vi "main_receiver_MIMO_OFDM.vi"() -> ()   [LabVIEW 2020] (continued)
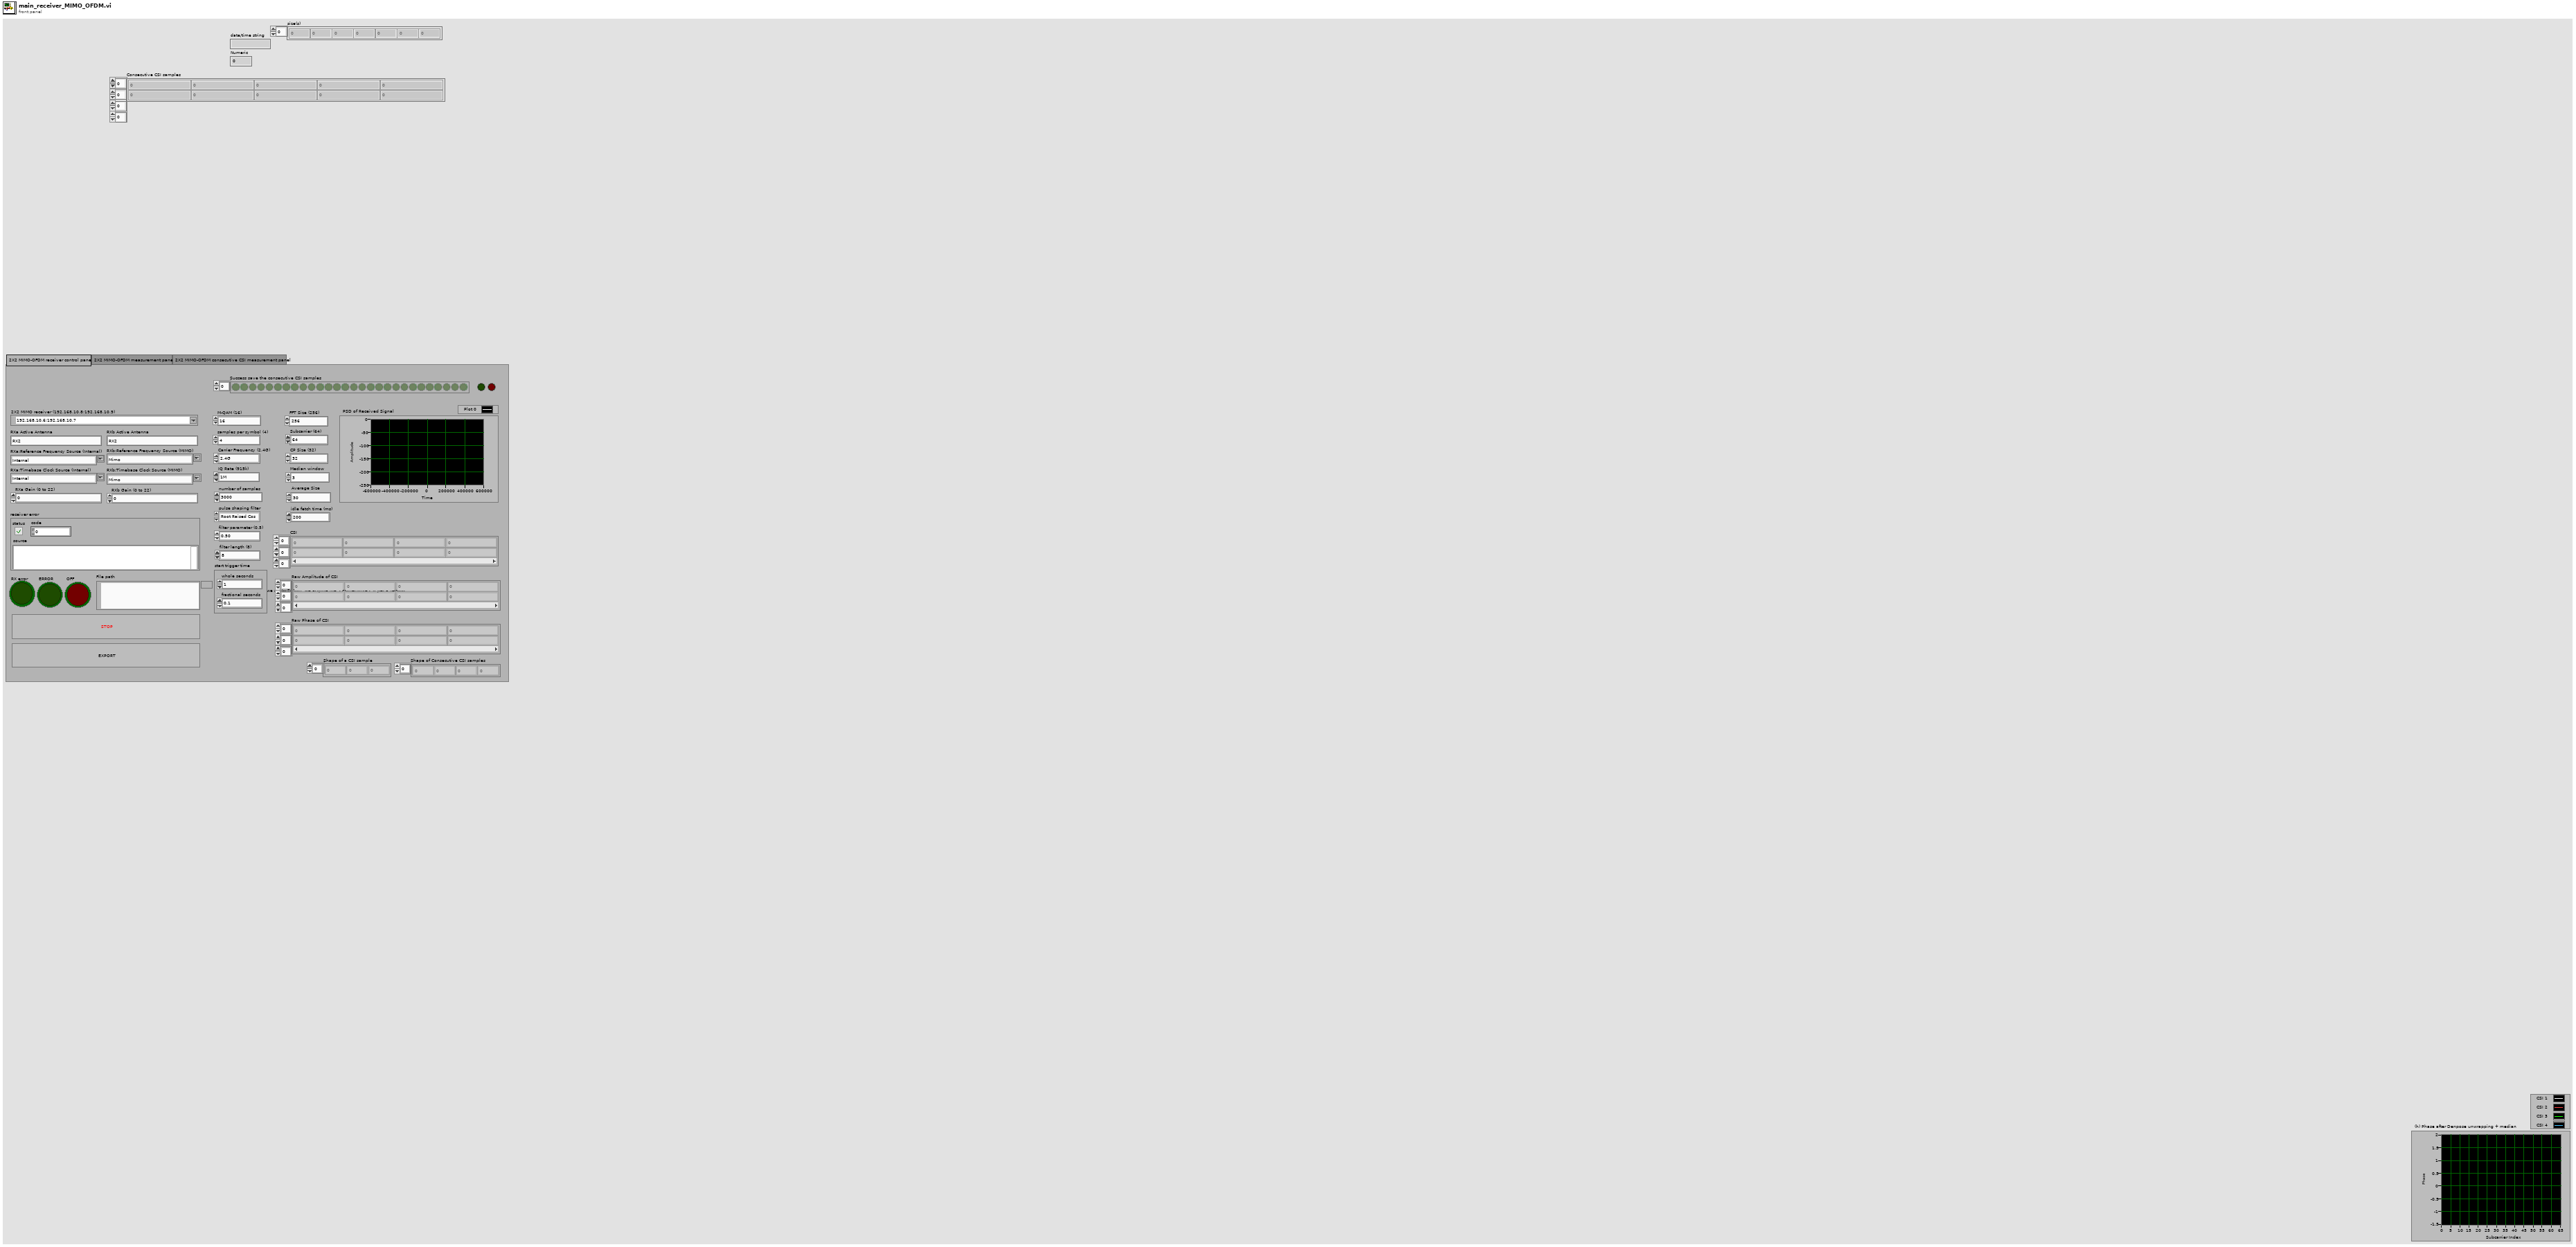
[diagram p1: front panel]
types:
  T1 = enum32{"2X2 MIMO-OFDM receiver control panel", "2X2 MIMO-OFDM measurement panel", "2X2 MIMO-OFDM consecutive CSI measurement panel"}
  T2 = typedef "niUSRP Timestamp.ctl" = cluster{"whole seconds":u64, "fractional seconds":dbl}
  T3 = enum16{"none", "Raised Cosine", "Root Raised Cos", "Gaussian"}
  T4 = enum16{"FSK", "PSK", "QAM", "MSK", "PAM", "ASK", "CPM"}
  T5 = cluster{"samples per symbol (16)":i32, "symbol map":cdb[]}
  T6 = typedef "niAMT.lvlib/Complex Data Waveform.ctl" = cluster{"t0":dbl, "dt":dbl, "Y":cdb[]}
  T7 = cluster{"f0":dbl, "df":dbl, "imaginary part":dbl[]}
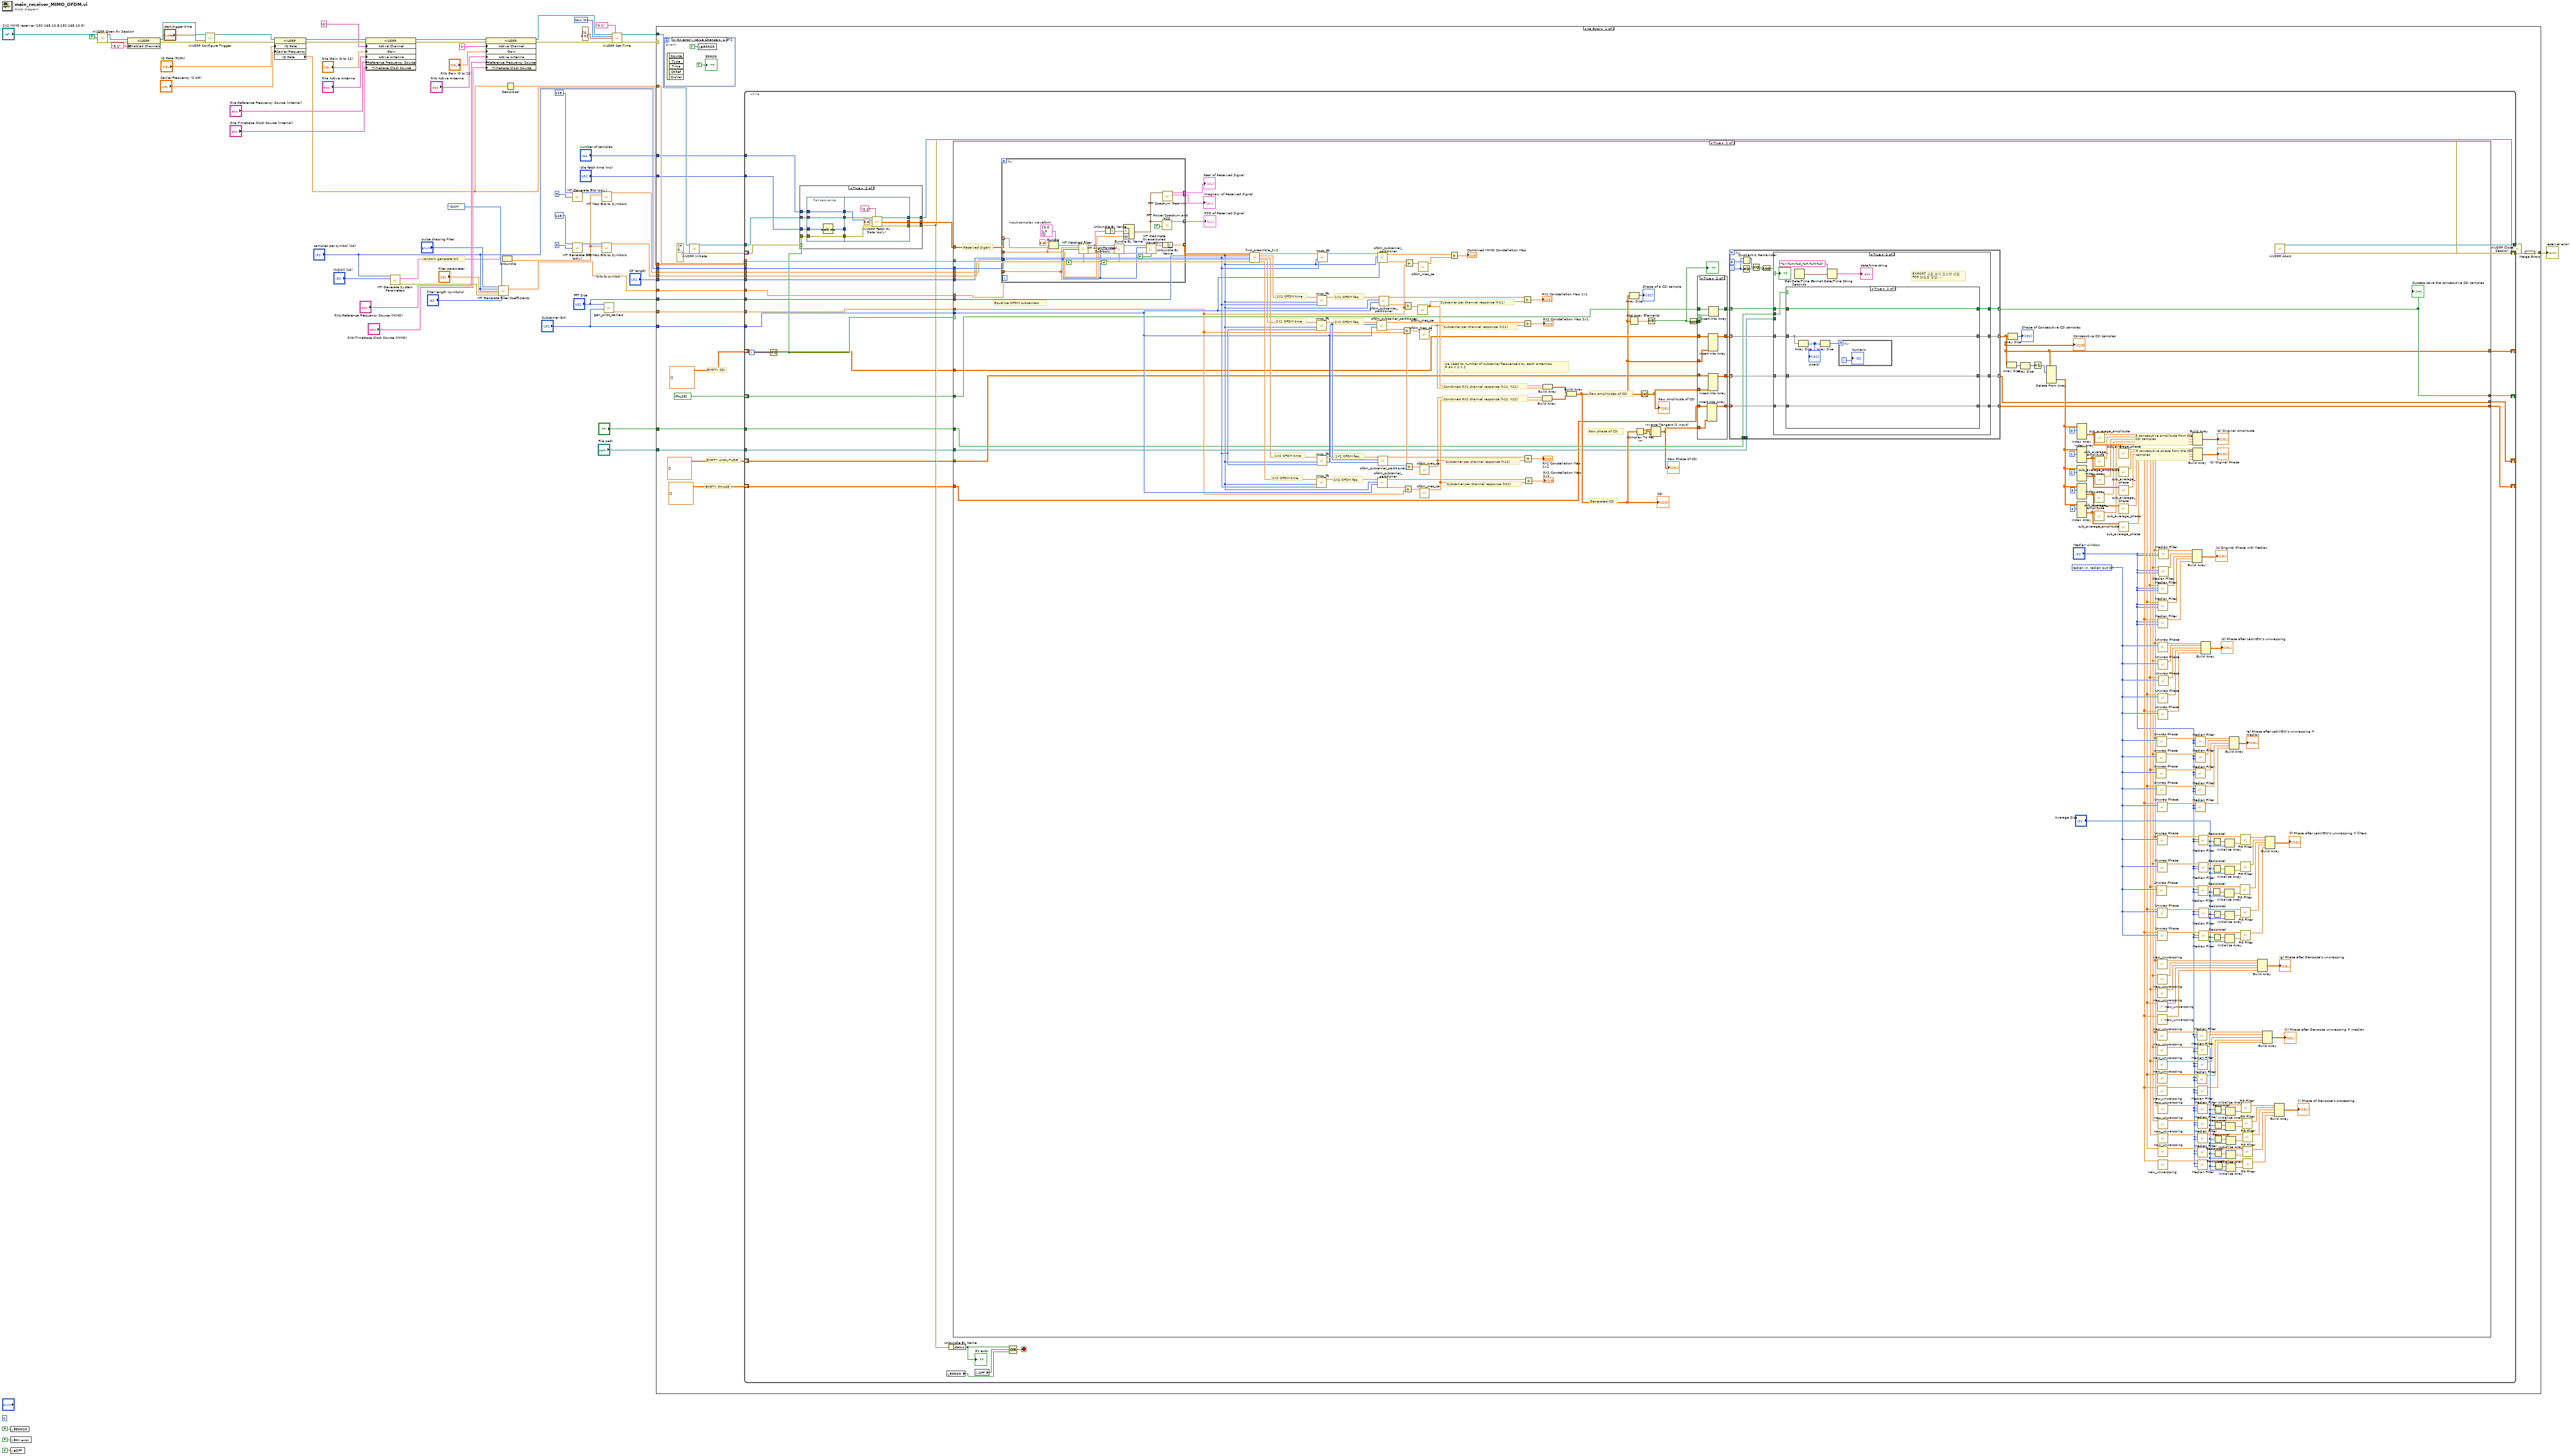
[diagram p0: block diagram]
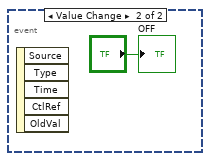
[diagram p2: hidden frame]
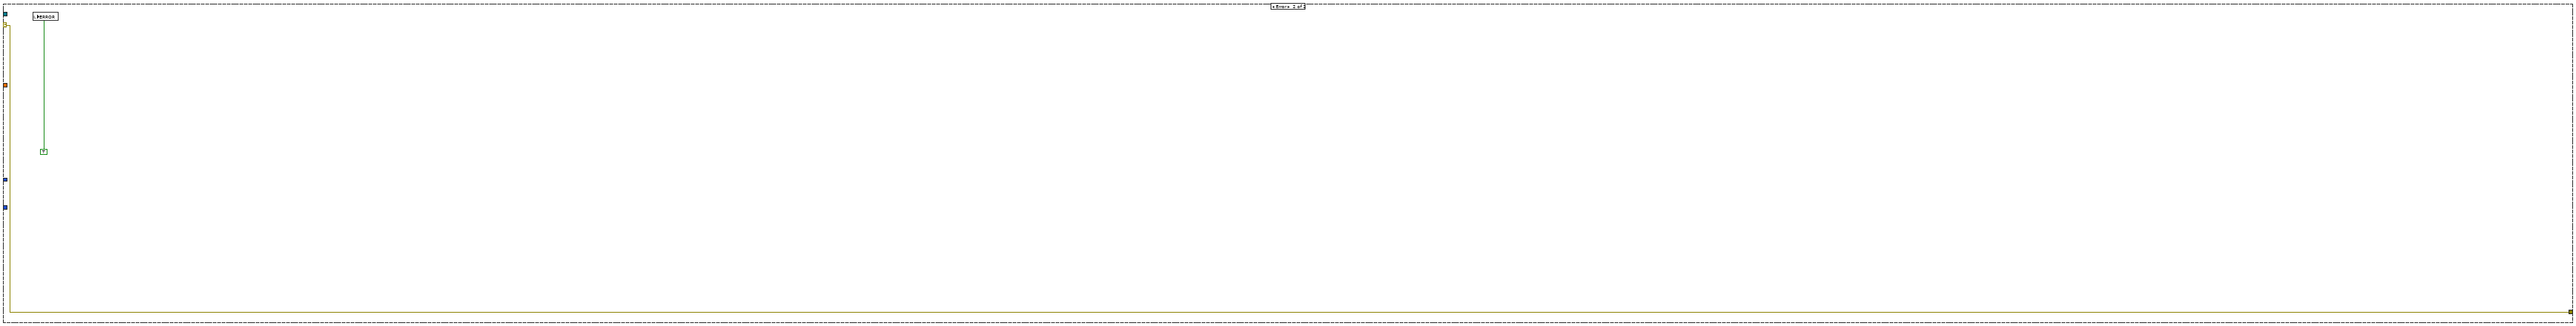
[diagram p8: hidden frame]
diagram:
  (unwired) 0 ("index")
  w44 = 0 items=["Now", "Next Timebase Edge"] ("apply timestamp")
  # "bits to symbol"
  # "random generate bit"
  n1 = local write "ERROR"(FALSE) -> ()
  n2 = local write "RX error"(FALSE) -> ()
  n3 = local write "OFF"(FALSE) -> ()
  n4 = call <instrlib>:"niUSRP Open Rx Session.vi"("device names"="2X2 MIMO receiver (192.168.10.8;192.168.10.9)", "reset"=TRUE) -> ("session handle out"=w32:refnum<k15>, "error out"=w31:errorcluster)  [unwired: 12 in]
  n5 = property class="niUSRP"(reference=w32, error in=w31, "Enabled Channels"="0,1" ("Configuration:Enabled Channels")) -> (reference out=w61:refnum<k15>, error out=w60:errorcluster)
  n6 = call-poly <instrlib>:"niUSRP Configure Trigger.vi"("session handle"=w61, "start trigger time"="start trigger time", "error in (no error)"=w60) -> ("session handle out"=w59:refnum<k15>, "error out"=w58:errorcluster)  [unwired: 11 in]
  n7 = property class="niUSRP"(reference=w59, error in=w58, "IQ Rate"="IQ Rate (915k)", "Carrier Frequency"="Carrier Frequency (2.4G)") -> (reference out=w57:refnum<k15>, error out=w56:errorcluster, "IQ Rate"=w6:dbl)
  n8 = property class="niUSRP"(reference=w57, error in=w56, "Active Channel"="0", "Gain"="RXa Gain (0 to 22)", "Active Antenna"="RXa Active Antenna", "Reference Frequency Source"="RXa:Reference Frequency Source (Internal)", "Timebase Clock Source"="RXa:Timebase Clock Source (Internal)") -> (reference out=w51:refnum<k15>, error out=w50:errorcluster)
  n9 = call-poly <vilib>:"MT Generate System Parameters.vi"("samples per symbol (16)"="samples per symbol (16)", "M-QAM (16)"="M-QAM (16)") -> ("QAM system parameters"=w19:T5, "error out"=w37:errorcluster)  [unwired: 11 in, 1 out]
  n10 = property class="niUSRP"(reference=w51, error in=w50, "Active Channel"="1", "Gain"="RXb Gain (0 to 22)", "Active Antenna"="RXb Active Antenna", "Reference Frequency Source"="RXb:Reference Frequency Source (MIMO)", "Timebase Clock Source"="RXb:Timebase Clock Source (MIMO)") -> (reference out=w30:refnum<k15>, error out=w9:errorcluster)
  n11 = call <vilib>:"MT Generate Filter Coefficients.vi"("pulse shaping filter (none)"="pulse shaping filter", "modulation type"=T4."QAM", "pulse shaping samples per symbol (16)"="samples per symbol (16)", "matched samples per symbol (16)"="samples per symbol (16)", "filter parameter"="filter parameter", "error in (no error)"=w37, "filter length (symbols)"="filter length (symbols)") -> ("matched filter coefficients"=w28:dbl[])  [unwired: 6 in, 2 out]
  n12 = Unbundle(w19) -> ("symbol map"=w14:cdb[])  [unwired: 1 out]
  n13 = Reciprocal(x=w6) -> (1/x=w35:dbl)
  n14 = call-poly <vilib>:"MT Generate Bits (poly).vi"("total bits (128)"=128, "PN sequence order (9)"=9) -> ("output bit stream"=w16:i8[])  [unwired: 11 in, 2 out]
  n15 = call-poly <vilib>:"MT Generate Bits (poly).vi"("total bits (128)"=128, "PN sequence order (9)"=5) -> ("output bit stream"=w18:i8[])  [unwired: 11 in, 2 out]
  n16 = call-poly <vilib>:"MT Map Bits to Symbols.vi"("input bit stream"=w16, "symbol map"=w14) -> ("symbols"=w10:cdb[])  [unwired: 12 in, 1 out]
  n17 = call-poly <vilib>:"MT Map Bits to Symbols.vi"("input bit stream"=w18, "symbol map"=w14) -> ("symbols"=w11:cdb[])  [unwired: 12 in, 1 out]
  n18 = call "gen_pilot_carriers.vi"("message carrier"="Subcarrier (64)", "FFT size"="FFT Size") -> ("RX pilot carriers"=w15:cdb[])  [unwired: 8 in, 1 out]
  n19 = call <instrlib>:"niUSRP Set Time.vi"("session handle"=w30, "channel list"="0,1" ("Configuration:Enabled Channels"), "apply timestamp"=w44, "timestamp"=T2 {"whole seconds"=0, "fractional seconds"=0.0}, "error in (no error)"=w9) -> ("session handle out"=w29:refnum<k15>, "error out"=w42:errorcluster)  [unwired: 9 in]
  n20 = case shown="No Error" w42 {
    selector: w42 -> [_ w434]
    tunnel: w29 -> [w84 _]
    tunnel: w35 -> [w87 _]
    tunnel: [w85 w434] -> w34
    tunnel: w28 -> [w82 _]
    tunnel: "samples per symbol (16)" -> [w81 _]
    tunnel: "FFT Size" -> [w80 _]
    tunnel: "Subcarrier (64)" -> [w79 _]
    tunnel: w10 -> [w78 _]
    tunnel: w11 -> [w77 _]
    tunnel: "CP length" -> [w76 _]
    tunnel: w15 -> [w75 _]
    tunnel: w6 -> [w74 _]
    tunnel: "number of samples" -> [w73 _]
    tunnel: "idle fetch time (ms)" -> [w72 _]
    tunnel: "?" -> [w69 _]
    tunnel: "File path" -> [w68 _]
    frame No Error {
      # "EMPTY PHASE"
      # "EMPTY AMPLITUDE"
      # "EMPTY CSI"
      n21 = event shown="[0] \"RX error\": Value Change" {
        selector: _ -> [_ _]
        dyn-events: _ -> [_ _]
        timeout: _ -> [_ _]
        event "RX error": Value Change {
          n22 = event-data() -> ()  [unwired: 1 in, 5 out]
          n23 = local write "ERROR"(TRUE) -> ()
          "ERROR" <- TRUE
        }
        event Value Change {
          n24 = event-data() -> ()  [unwired: 1 in, 5 out]
          "OFF" <- "?"
        }
      }
      n25 = call <instrlib>:"niUSRP Initiate.vi"("session handle"=w84, "error in (no error)"=errorcluster {"status"=FALSE, "code"=0, "source"=""}) -> ("session handle out"=w93:refnum<k15>, "error out"=w92:errorcluster)  [unwired: 12 in]
      n26 = while {
        tunnel: w93 -> [w115]
        shift-right: [w111] -> w91
        shift-left: w92 -> [w110]
        tunnel: [w113] -> w90
        tunnel: w87 -> [w128]
        tunnel: w82 -> [w125]
        tunnel: w81 -> [w124]
        tunnel: w80 -> [w121]
        tunnel: w79 -> [w120]
        tunnel: w78 -> [w119]
        tunnel: w77 -> [w118]
        tunnel: w76 -> [w117]
        tunnel: w75 -> [w116]
        tunnel: w74 -> [_]
        tunnel: w73 -> [w114]
        tunnel: w72 -> [w109]
        shift-right: [w103] -> _
        shift-left: cdb[][][][] [] ("appended array") -> [w106]
        shift-right: [w104] -> _
        shift-left: bool[] [FALSE] ("Received CSI 3") -> [w105]
        tunnel: w69 -> [w102]
        tunnel: w68 -> [w101]
        shift-right: [w98] -> _
        shift-left: cdb[][][][] [] ("appended array") -> [w100]
        shift-right: [w97] -> _
        shift-left: cdb[][][][] [] ("appended array") -> [w99]
        i -> [w108]
        stop <- w126 stop-if-true
        n27 = Not Equal To 0?(x=w108) -> (x != 0?=w107:bool)
        n28 = case shown="True" w107 {
          tunnel: w115 -> [w130 w141]
          tunnel: w114 -> [_ w136]
          tunnel: [w130 w139] -> w113
          tunnel: [_ w137] -> w112
          tunnel: [w129 w138] -> w111
          tunnel: w110 -> [w129 w134]
          tunnel: w109 -> [_ w132]
          frame False {
          }
          frame True {
            n29 = flat-sequence {
              tunnel: w141 -> [w146]
              tunnel: [w146] -> w140
              tunnel: w136 -> [w145]
              tunnel: [w145] -> w135
              tunnel: w134 -> [w144]
              tunnel: [w144] -> w133
              tunnel: w132 -> [w143]
              tunnel: [w142] -> w131
              tunnel: w140 -> [w154]
              tunnel: [w153] -> w139
              tunnel: [w152] -> w138
              tunnel: [w151] -> w137
              tunnel: w135 -> [w150]
              tunnel: w133 -> [w147]
              tunnel: w131 -> [_]
              frame #0 {
                n30 = Wait (ms)(milliseconds to wait=w143) -> (millisecond timer value=w142:u32)
              }
              frame #1 {
                n31 = call-poly <instrlib>:"niUSRP Fetch Rx Data (poly).vi"("session handle"=w154, "channel list"="0,1", "number of samples"=w150, "timeout"=3.0, "error in (no error)"=w147) -> ("session handle out"=w153:refnum<k15>, "data"=w151:cdb[][], "error out"=w152:errorcluster)  [unwired: 7 in, 1 out]
              }
            }
          }
        }
        n32 = local read "ERROR"() -> (w123:bool)
        n33 = Unbundle By Name(w111) -> ("status"=w127:bool)
        "RX error" <- w127
        n34 = case shown="True" w107 {
          tunnel: w112 -> [_ w346]
          tunnel: w128 -> [_ w350]
          tunnel: w125 -> [_ w349]
          tunnel: w124 -> [_ w348]
          tunnel: w121 -> [_ w303]
          tunnel: w120 -> [_ w302]
          tunnel: w119 -> [_ w345]
          tunnel: w118 -> [_ w347]
          tunnel: w117 -> [_ w305]
          tunnel: w116 -> [_ w299]
          tunnel: w106 -> [_ w293]
          tunnel: w105 -> [_ w294]
          tunnel: [_ w283] -> w104
          tunnel: [_ w282] -> w103
          tunnel: w102 -> [_ w164]
          tunnel: w101 -> [_ w163]
          tunnel: w100 -> [_ w162]
          tunnel: w99 -> [_ w160]
          tunnel: [_ w156] -> w98
          tunnel: [_ w155] -> w97
          frame False {
          }
          frame True {
            w216 = 0 items=["radian in, radian out", "radian in, degree out", "degree in, degree out", "degree in, radian out"] ("phase unit")
            # "5 consecutive phase from the CSI samples"
            # "5 consecutive amplitude from the CSI samples"
            # "Raw phase of CSI"
            # "Raw amplitudes of CSI"
            # "Generated CSI"
            # "Combined RX2 channel response (h12, h22)"
            # "Combined RX1 channel response (h11, h21)"
            # "Subcarrier per channel response (h22)"
            # "Subcarrier per channel response (h21)"
            # "Subcarrier per channel response (h12)"
            # "Subcarrier per channel response (h11)"
            # "2X2 OFDM feq."
            # "2X1 OFDM feq."
            # "1X2 OFDM feq."
            # "1X1 OFDM feq."
            # "2X2 OFDM time"
            # "2X1 OFDM time"
            # "1X2 OFDM time"
            # "1X1 OFDM time"
            # "we need to number of subcarrier frequenceis by each antennas\n= 64 X 2 X 2"
            # "Received Siganl"
            # "Equalize OFDM subcarriers"
            n35 = for {
              tunnel: w350 -> [w430]
              tunnel: w346 -> [w416] mode=indexing
              tunnel: w349 -> [w426]
              tunnel: w348 -> [w423]
              tunnel: [w415] -> w295 mode=indexing
              tunnel: [w413] -> w315 mode=indexing
              tunnel: [w412] -> w314 mode=indexing
              tunnel: [w411] -> w313 mode=indexing
              w431 = T6 {"t0"=0.0, "dt"=1.0, "Y"=[]}  # input complex waveform
              n36 = Bundle(cluster=w431, "t0"=0.0, "dt"=w430, "Y"=w416) -> (w428:T6)
              n37 = call-poly <vilib>:"MT Matched Filter.vi"("input complex waveform"=w428, "matched filter coefficients"=w426, "samples per symbol (16)"=w423, "reset? (T)"=FALSE) -> ("output complex waveform"=w427:T6, "error out"=w425:errorcluster)  [unwired: 10 in]
              n38 = Unbundle By Name(w427) -> ("Y"=w418:cdb[])
              n39 = call-poly <vilib>:"MT Align To Ideal Symbols.vi"("input complex waveform"=w427, "matched filter coefficients"=w426, "samples per symbol (16)"=w423, "error in (no error)"=w425, "reset? (T)"=FALSE) -> ("output complex waveform"=w417:T6, "error out"=w424:errorcluster)  [unwired: 8 in, 1 out]
              n40 = Bundle By Name("Y"=w418, "dt"=w430) -> (w414:waveform(cdb))  [unwired: 1 in]
              n41 = call <vilib>:"MT Decimate Oversampled Waveform.vi"("input complex waveform"=w417, "decimation factor"=w423, "error in (no error)"=w424, "reset? (T)"=FALSE) -> ("output complex waveform"=w422:T6)  [unwired: 10 in, 1 out]
              n42 = call-poly <vilib>:"FFT Power Spectrum and PSD.vi"("dB On (F)"=TRUE, "time signal"=w414) -> ("Power Spectrum / PSD"=w413:cluster{"f0":dbl, "df":dbl, "magnitude":dbl[]})  [unwired: 6 in, 3 out]
              n43 = call-poly <vilib>:"FFT Spectrum (Real-Im).vi"("time signal"=w414) -> ("imaginary part"=w411:T7, "real part"=w412:cluster{"f0":dbl, "df":dbl, "real part":dbl[]})  [unwired: 6 in, 3 out]
              n44 = Unbundle By Name(w422) -> ("Y"=w415:cdb[])
            }
            "PSD of Received Signal" <- w315
            "Real of Received Signal" <- w314
            "Imagnary of Received Signal" <- w313
            n45 = call "find_preamble_2x2.vi"("received \ntime symbol"=w295, "FFT Size"=w303, "CP Length"=w305, "1st preamble"=w345, "2nd preamble"=w347) -> ("Received OFDM symbol (vector)"=w306:cdb[], "Received OFDM symbol (h11)"=w328:cdb[], "Received OFDM symbol (h12)"=w321:cdb[], "Received OFDM symbol (h21)"=w327:cdb[], "Received OFDM symbol (h22)"=w326:cdb[])  [unwired: 6 in]
            n46 = call "rmcp_fft.vi"("CP length"=w305, "fft size"=w303, "time symbol"=w327) -> ("freq output"=w342:cdb[])  [unwired: 8 in]
            n47 = call "rmcp_fft.vi"("CP length"=w305, "fft size"=w303, "time symbol"=w326) -> ("freq output"=w341:cdb[])  [unwired: 8 in]
            n48 = call "rmcp_fft.vi"("CP length"=w305, "fft size"=w303, "time symbol"=w328) -> ("freq output"=w344:cdb[])  [unwired: 8 in]
            n49 = call "rmcp_fft.vi"("CP length"=w305, "fft size"=w303, "time symbol"=w321) -> ("freq output"=w343:cdb[])  [unwired: 8 in]
            n50 = call "rmcp_fft.vi"("CP length"=w305, "fft size"=w303, "time symbol"=w306) -> ("freq output"=w304:cdb[])  [unwired: 8 in]
            n51 = call "ofdm_subcarrier_partitioner.vi"("message carrier"=w302, "FFT size"=w303, "received symbol"=w342) -> ("pilot subcarriers"=w338:cdb[], "message subcarriers"=w332:cdb[])  [unwired: 7 in]
            n52 = call "ofdm_subcarrier_partitioner.vi"("message carrier"=w302, "FFT size"=w303, "received symbol"=w341) -> ("pilot subcarriers"=w337:cdb[], "message subcarriers"=w330:cdb[])  [unwired: 7 in]
            n53 = call "ofdm_subcarrier_partitioner.vi"("message carrier"=w302, "FFT size"=w303, "received symbol"=w304) -> ("pilot subcarriers"=w300:cdb[], "message subcarriers"=w298:cdb[])  [unwired: 7 in]
            n54 = call "ofdm_subcarrier_partitioner.vi"("message carrier"=w302, "FFT size"=w303, "received symbol"=w343) -> ("pilot subcarriers"=w339:cdb[], "message subcarriers"=w334:cdb[])  [unwired: 7 in]
            n55 = call "ofdm_subcarrier_partitioner.vi"("message carrier"=w302, "FFT size"=w303, "received symbol"=w344) -> ("pilot subcarriers"=w340:cdb[], "message subcarriers"=w336:cdb[])  [unwired: 7 in]
            n56 = Divide(x=w338, y=w299) -> (x/y=w324:cdb[])
            n57 = Divide(x=w340, y=w299) -> (x/y=w322:cdb[])
            n58 = Divide(x=w337, y=w299) -> (x/y=w323:cdb[])
            n59 = Divide(x=w339, y=w299) -> (x/y=w325:cdb[])
            n60 = Divide(x=w300, y=w299) -> (x/y=w301:cdb[])
            n61 = call "ofdm_mes_ce.vi"("ZF \nchannel \nestimates"=w322) -> ("interpolated\n mes carrier CE"=w319:cdb[])  [unwired: 8 in, 2 out]
            n62 = call "ofdm_mes_ce.vi"("ZF \nchannel \nestimates"=w301) -> ("interpolated\n mes carrier CE"=w291:cdb[])  [unwired: 8 in, 2 out]
            n63 = call "ofdm_mes_ce.vi"("ZF \nchannel \nestimates"=w324) -> ("interpolated\n mes carrier CE"=w318:cdb[])  [unwired: 8 in, 2 out]
            n64 = call "ofdm_mes_ce.vi"("ZF \nchannel \nestimates"=w325) -> ("interpolated\n mes carrier CE"=w317:cdb[])  [unwired: 8 in, 2 out]
            n65 = call "ofdm_mes_ce.vi"("ZF \nchannel \nestimates"=w323) -> ("interpolated\n mes carrier CE"=w316:cdb[])  [unwired: 8 in, 2 out]
            n66 = Divide(x=w298, y=w291) -> (x/y=→"Combined MIMO Constellation Map":cdb[])
            n67 = Divide(x=w336, y=w319) -> (x/y=→"RX1 Constellation Map 1x1":cdb[])
            n68 = Divide(x=w332, y=w318) -> (x/y=→"RX2 Constellation Map 2x1":cdb[])
            n69 = Divide(x=w334, y=w317) -> (x/y=→"RX1 Constellation Map 1x2":cdb[])
            n70 = Divide(x=w330, y=w316) -> (x/y=→"RX2 Constellation Map 2x2":cdb[])
            n71 = Build Array(w317, w316) -> (w320:cdb[][])
            n72 = Build Array "Build Array"(w319, w318) -> (w290:cdb[][])
            n73 = Build Array "Build Array"(w290, w320) -> (w288:cdb[][][])
            "CSI" <- w288
            n74 = Add Array Elements(numeric array=w288) -> (sum=w296:cdb)
            n75 = Array Size(array=w288) -> (size(s)=→"Shape of a CSI sample":i32[])
            n76 = Complex To Re/Im(x + iy=w288) -> (x=w311:dbl[][][], y=w312:dbl[][][])
            n77 = Absolute Value ("Absolute Value.vi")(x=w288) -> (abs(x)=w161:dbl[][][])
            "Raw Amplitude of CSI" <- w161
            n78 = Equal To 0?(x=w296) -> (x = 0?=w287:bool)
            "?" <- w287
            n79 = Inverse Tangent (2 Input)(1:w311, 2:w312) -> (0:w159:dbl[][][])
            "Raw Phase of CSI" <- w159
            n80 = Not(x=w287) -> (.not. x?=w286:bool)
            n81 = case shown="True" w286 {
              tunnel: w286 -> [_ w410]
              tunnel: w294 -> [w397 w407]
              tunnel: [w397 w405] -> w284
              tunnel: w288 -> [_ w409]
              tunnel: w293 -> [w398 w408]
              tunnel: [w398 w406] -> w285
              tunnel: w162 -> [w396 w404]
              tunnel: w161 -> [_ w403]
              tunnel: w160 -> [w395 w402]
              tunnel: w159 -> [_ w401]
              tunnel: [w396 w400] -> w158
              tunnel: [w395 w399] -> w157
              frame False {
              }
              frame True {
                n82 = Insert Into Array(array=w402, new element=w401) -> (w399:cdb[][][][])  [unwired: 4 in]
                n83 = Insert Into Array(array=w408, new element=w409) -> (w406:cdb[][][][])  [unwired: 4 in]
                n84 = Insert Into Array(array=w404, new element=w403) -> (w400:cdb[][][][])  [unwired: 4 in]
                n85 = Insert Into Array(array=w407, new element=w410) -> (w405:bool[])  [unwired: 1 in]
              }
            }
            n86 = for {
              tunnel: w285 -> [w360] mode=indexing
              tunnel: [w359] -> w282 mode=indexing
              tunnel: w284 -> [w362] mode=indexing
              tunnel: [w361] -> w283 mode=indexing
              tunnel: w164 -> [w356]
              tunnel: w163 -> [w355]
              tunnel: w158 -> [w354] mode=indexing
              tunnel: w157 -> [w353] mode=indexing
              tunnel: [w352] -> w156 mode=indexing
              tunnel: [w351] -> w155 mode=indexing
              i -> [w357]
              n87 = Not Equal To 0?(x=w357) -> (x != 0?=w366:bool)
              n88 = Quotient & Remainder(x=w357, y=5) -> (x-y*floor(x/y)=w364:i32)  [unwired: 1 out]
              n89 = Equal To 0?(x=w364) -> (x = 0?=w363:bool)
              n90 = And(x=w363, y=w366) -> (x .and. y?=w358:bool)
              n91 = case shown="True" w358 {
                selector: w358 -> [_ w383]
                tunnel: w362 -> [w370 w378]
                tunnel: [w370 w377] -> w361
                tunnel: w360 -> [w369 w376]
                tunnel: [w369 w375] -> w359
                tunnel: w356 -> [_ w379]
                tunnel: w355 -> [_ _]
                tunnel: w354 -> [w368 w374]
                tunnel: w353 -> [w367 w372]
                tunnel: [w368 w373] -> w352
                tunnel: [w367 w371] -> w351
                frame False {
                }
                frame True {
                  # "EXPORT 구문 여기 있으면 안됨\nFOR 탈출을 못함...."
                  n92 = case shown="True" w379 {
                    tunnel: w378 -> [w387 w393]
                    tunnel: [w387 w393] -> w377
                    tunnel: w376 -> [w386 w390]
                    tunnel: [w386 w390] -> w375
                    tunnel: w374 -> [w385 w391]
                    tunnel: [w385 w391] -> w373
                    tunnel: w372 -> [w384 w392]
                    tunnel: [w384 w392] -> w371
                    frame False {
                    }
                    frame True {
                      n93 = Array Size(array=w390) -> (size(s)=w389:i32[])
                      "size(s)" <- w389
                      n94 = Array Size(array=w389) -> (size(s)=w388:i32)
                      n95 = for {
                        N: w388 -> [_]
                        i -> [w394]
                        "Numeric" <- w394
                      }
                    }
                  }
                  n96 = Get Date/Time In Seconds() -> (seconds since 1Jan1904=w382:timestamp)
                  n97 = Format Date/Time String(time format string (%c)="%Y-%m-%d_%H-%M-%S", seconds (now)=w382) -> (date/time string=→"date/time string":string)  [unwired: 1 in]
                  "?" <- w383
                }
              }
            }
            "Consecutive CSI samples" <- w282
            "Success save the consecutive CSI samples" <- w283
            n98 = Array Size(array=w282) -> (size(s)=w281:i32[])
            n99 = Array Size(array=w282) -> (size(s)=→"Shape of Consecutive CSI samples":i32[])
            n100 = Array Size(array=w281) -> (size(s)=w280:i32)
            n101 = Increment(x=w280) -> (x+1=w279:i32)
            n102 = Delete From Array "Delete From Array"(array=w282, length=w279) -> (deleted portion=w277:cdb[][][][])  [unwired: 4 in, 1 out]
            n103 = Index Array(array=w277, index (dim 0)=0 ("index (vol)")) -> (element=w272:cdb[][][])  [unwired: 3 in]
            n104 = Index Array(array=w277, index (dim 0)=1 ("index (vol)")) -> (element=w271:cdb[][][])  [unwired: 3 in]
            n105 = Index Array(array=w277, index (dim 0)=2 ("index (vol)")) -> (element=w270:cdb[][][])  [unwired: 3 in]
            n106 = Index Array(array=w277, index (dim 0)=3 ("index (vol)")) -> (element=w269:cdb[][][])  [unwired: 3 in]
            n107 = Index Array(array=w277, index (dim 0)=4 ("index (vol)")) -> (element=w262:cdb[][][])  [unwired: 3 in]
            n108 = call "sub_average_amplitude.vi"("Input CSI sample"=w262) -> ("Array"=w264:dbl[])  [unwired: 10 in]
            n109 = call "sub_average_amplitude.vi"("Input CSI sample"=w269) -> ("Array"=w265:dbl[])  [unwired: 10 in]
            n110 = call "sub_average_amplitude.vi"("Input CSI sample"=w271) -> ("Array"=w267:dbl[])  [unwired: 10 in]
            n111 = call "sub_average_amplitude.vi"("Input CSI sample"=w270) -> ("Array"=w266:dbl[])  [unwired: 10 in]
            n112 = call "sub_average_amplitude.vi"("Input CSI sample"=w272) -> ("Array"=w268:dbl[])  [unwired: 10 in]
            n113 = call "sub_average_phase.vi"("Input CSI sample"=w271) -> ("Array"=w169:dbl[])  [unwired: 10 in]
            n114 = call "sub_average_phase.vi"("Input CSI sample"=w262) -> ("Array"=w166:dbl[])  [unwired: 10 in]
            n115 = call "sub_average_phase.vi"("Input CSI sample"=w272) -> ("Array"=w170:dbl[])  [unwired: 10 in]
            n116 = call "sub_average_phase.vi"("Input CSI sample"=w270) -> ("Array"=w168:dbl[])  [unwired: 10 in]
            n117 = call "sub_average_phase.vi"("Input CSI sample"=w269) -> ("Array"=w167:dbl[])  [unwired: 10 in]
            n118 = call <vilib>:"Unwrap Phase.vi"("phase unit"=w216, "Phase"=w169) -> ("Unwrapped Phase"=w248:dbl[])  [unwired: 8 in, 1 out]
            n119 = call <vilib>:"Unwrap Phase.vi"("phase unit"=w216, "Phase"=w168) -> ("Unwrapped Phase"=w247:dbl[])  [unwired: 8 in, 1 out]
            n120 = call <vilib>:"Unwrap Phase.vi"("phase unit"=w216, "Phase"=w167) -> ("Unwrapped Phase"=w246:dbl[])  [unwired: 8 in, 1 out]
            n121 = call <vilib>:"Unwrap Phase.vi"("phase unit"=w216, "Phase"=w170) -> ("Unwrapped Phase"=w249:dbl[])  [unwired: 8 in, 1 out]
            n122 = call <vilib>:"Unwrap Phase.vi"("phase unit"=w216, "Phase"=w168) -> ("Unwrapped Phase"=w237:dbl[])  [unwired: 8 in, 1 out]
            n123 = call <vilib>:"Unwrap Phase.vi"("phase unit"=w216, "Phase"=w166) -> ("Unwrapped Phase"=w245:dbl[])  [unwired: 8 in, 1 out]
            n124 = call <vilib>:"Unwrap Phase.vi"("phase unit"=w216, "Phase"=w170) -> ("Unwrapped Phase"=w308:dbl[])  [unwired: 8 in, 1 out]
            n125 = call <vilib>:"Unwrap Phase.vi"("phase unit"=w216, "Phase"=w169) -> ("Unwrapped Phase"=w241:dbl[])  [unwired: 8 in, 1 out]
            n126 = call <vilib>:"Unwrap Phase.vi"("phase unit"=w216, "Phase"=w167) -> ("Unwrapped Phase"=w233:dbl[])  [unwired: 8 in, 1 out]
            n127 = call <vilib>:"Unwrap Phase.vi"("phase unit"=w216, "Phase"=w166) -> ("Unwrapped Phase"=w229:dbl[])  [unwired: 8 in, 1 out]
            n128 = call "new_unwarpping.vi"("phase"=w170) -> ("unwrapped_phase"=w215:dbl[])  [unwired: 10 in]
            n129 = call "new_unwarpping.vi"("phase"=w169) -> ("unwrapped_phase"=w214:dbl[])  [unwired: 10 in]
            n130 = call "new_unwarpping.vi"("phase"=w168) -> ("unwrapped_phase"=w213:dbl[])  [unwired: 10 in]
            n131 = call "new_unwarpping.vi"("phase"=w167) -> ("unwrapped_phase"=w212:dbl[])  [unwired: 10 in]
            n132 = call "new_unwarpping.vi"("phase"=w166) -> ("unwrapped_phase"=w211:dbl[])  [unwired: 10 in]
            n133 = call "new_unwarpping.vi"("phase"=w170) -> ("unwrapped_phase"=w208:dbl[])  [unwired: 10 in]
            n134 = call "new_unwarpping.vi"("phase"=w169) -> ("unwrapped_phase"=w207:dbl[])  [unwired: 10 in]
            n135 = call "new_unwarpping.vi"("phase"=w168) -> ("unwrapped_phase"=w206:dbl[])  [unwired: 10 in]
            n136 = call "new_unwarpping.vi"("phase"=w167) -> ("unwrapped_phase"=w205:dbl[])  [unwired: 10 in]
            n137 = call "new_unwarpping.vi"("phase"=w166) -> ("unwrapped_phase"=w204:dbl[])  [unwired: 10 in]
            n138 = call <vilib>:"Unwrap Phase.vi"("phase unit"=w216, "Phase"=w166) -> ("Unwrapped Phase"=w218:dbl[])  [unwired: 8 in, 1 out]
            n139 = call "new_unwarpping.vi"("phase"=w170) -> ("unwrapped_phase"=w197:dbl[])  [unwired: 10 in]
            n140 = call "new_unwarpping.vi"("phase"=w169) -> ("unwrapped_phase"=w196:dbl[])  [unwired: 10 in]
            n141 = call "new_unwarpping.vi"("phase"=w168) -> ("unwrapped_phase"=w195:dbl[])  [unwired: 10 in]
            n142 = call "new_unwarpping.vi"("phase"=w167) -> ("unwrapped_phase"=w194:dbl[])  [unwired: 10 in]
            n143 = call "new_unwarpping.vi"("phase"=w166) -> ("unwrapped_phase"=w193:dbl[])  [unwired: 10 in]
            n144 = call <vilib>:"Median Filter.vi"("right rank"="Median window", "left rank"="Median window", "X"=w168) -> ("Filtered X"=w258:dbl[])  [unwired: 7 in, 1 out]
            n145 = call <vilib>:"Median Filter.vi"("right rank"="Median window", "left rank"="Median window", "X"=w167) -> ("Filtered X"=w257:dbl[])  [unwired: 7 in, 1 out]
            n146 = call <vilib>:"Median Filter.vi"("right rank"="Median window", "left rank"="Median window", "X"=w166) -> ("Filtered X"=w256:dbl[])  [unwired: 7 in, 1 out]
            n147 = call <vilib>:"Unwrap Phase.vi"("phase unit"=w216, "Phase"=w170) -> ("Unwrapped Phase"=w222:dbl[])  [unwired: 8 in, 1 out]
            n148 = call <vilib>:"Unwrap Phase.vi"("phase unit"=w216, "Phase"=w169) -> ("Unwrapped Phase"=w221:dbl[])  [unwired: 8 in, 1 out]
            n149 = call <vilib>:"Unwrap Phase.vi"("phase unit"=w216, "Phase"=w167) -> ("Unwrapped Phase"=w219:dbl[])  [unwired: 8 in, 1 out]
            n150 = call <vilib>:"Median Filter.vi"("right rank"="Median window", "left rank"="Median window", "X"=w170) -> ("Filtered X"=w260:dbl[])  [unwired: 7 in, 1 out]
            n151 = call <vilib>:"Median Filter.vi"("right rank"="Median window", "left rank"="Median window", "X"=w169) -> ("Filtered X"=w259:dbl[])  [unwired: 7 in, 1 out]
            n152 = call <vilib>:"Unwrap Phase.vi"("phase unit"=w216, "Phase"=w168) -> ("Unwrapped Phase"=w220:dbl[])  [unwired: 8 in, 1 out]
            n153 = Build Array(w260, w259, w258, w257, w256) -> (→"(c) Original Phase with Median":dbl[][])
            n154 = Build Array(w268, w267, w266, w265, w264) -> (→"(a) Original Amplitude":dbl[][])
            n155 = Build Array(w170, w169, w168, w167, w166) -> (→"(b) Orginal Phase":dbl[][])
            n156 = call <vilib>:"Median Filter.vi"("right rank"="Median window", "left rank"="Median window", "X"=w247) -> ("Filtered X"=w252:dbl[])  [unwired: 7 in, 1 out]
            n157 = call <vilib>:"Median Filter.vi"("right rank"="Median window", "left rank"="Median window", "X"=w246) -> ("Filtered X"=w251:dbl[])  [unwired: 7 in, 1 out]
            n158 = call <vilib>:"Median Filter.vi"("right rank"="Median window", "left rank"="Median window", "X"=w245) -> ("Filtered X"=w250:dbl[])  [unwired: 7 in, 1 out]
            n159 = call <vilib>:"Median Filter.vi"("right rank"="Median window", "left rank"="Median window", "X"=w249) -> ("Filtered X"=w254:dbl[])  [unwired: 7 in, 1 out]
            n160 = call <vilib>:"Median Filter.vi"("right rank"="Median window", "left rank"="Median window", "X"=w248) -> ("Filtered X"=w253:dbl[])  [unwired: 7 in, 1 out]
            n161 = call <vilib>:"Median Filter.vi"("right rank"="Median window", "left rank"="Median window", "X"=w208) -> ("Filtered X"=w203:dbl[])  [unwired: 7 in, 1 out]
            n162 = call <vilib>:"Median Filter.vi"("right rank"="Median window", "left rank"="Median window", "X"=w205) -> ("Filtered X"=w200:dbl[])  [unwired: 7 in, 1 out]
            n163 = call <vilib>:"Median Filter.vi"("right rank"="Median window", "left rank"="Median window", "X"=w207) -> ("Filtered X"=w202:dbl[])  [unwired: 7 in, 1 out]
            n164 = call <vilib>:"Median Filter.vi"("right rank"="Median window", "left rank"="Median window", "X"=w206) -> ("Filtered X"=w201:dbl[])  [unwired: 7 in, 1 out]
            n165 = call <vilib>:"Median Filter.vi"("right rank"="Median window", "left rank"="Median window", "X"=w204) -> ("Filtered X"=w199:dbl[])  [unwired: 7 in, 1 out]
            n166 = call <vilib>:"Median Filter.vi"("right rank"="Median window", "left rank"="Median window", "X"=w197) -> ("Filtered X"=w181:dbl[])  [unwired: 7 in, 1 out]
            n167 = call <vilib>:"Median Filter.vi"("right rank"="Median window", "left rank"="Median window", "X"=w194) -> ("Filtered X"=w178:dbl[])  [unwired: 7 in, 1 out]
            n168 = call <vilib>:"Median Filter.vi"("right rank"="Median window", "left rank"="Median window", "X"=w196) -> ("Filtered X"=w180:dbl[])  [unwired: 7 in, 1 out]
            n169 = call <vilib>:"Median Filter.vi"("right rank"="Median window", "left rank"="Median window", "X"=w195) -> ("Filtered X"=w179:dbl[])  [unwired: 7 in, 1 out]
            n170 = call <vilib>:"Median Filter.vi"("right rank"="Median window", "left rank"="Median window", "X"=w193) -> ("Filtered X"=w177:dbl[])  [unwired: 7 in, 1 out]
            n171 = call <vilib>:"Median Filter.vi"("right rank"="Median window", "left rank"="Median window", "X"=w237) -> ("Filtered X"=w236:dbl[])  [unwired: 7 in, 1 out]
            n172 = call <vilib>:"Median Filter.vi"("right rank"="Median window", "left rank"="Median window", "X"=w308) -> ("Filtered X"=w307:dbl[])  [unwired: 7 in, 1 out]
            n173 = call <vilib>:"Median Filter.vi"("right rank"="Median window", "left rank"="Median window", "X"=w241) -> ("Filtered X"=w240:dbl[])  [unwired: 7 in, 1 out]
            n174 = call <vilib>:"Median Filter.vi"("right rank"="Median window", "left rank"="Median window", "X"=w233) -> ("Filtered X"=w232:dbl[])  [unwired: 7 in, 1 out]
            n175 = call <vilib>:"Median Filter.vi"("right rank"="Median window", "left rank"="Median window", "X"=w229) -> ("Filtered X"=w228:dbl[])  [unwired: 7 in, 1 out]
            n176 = Build Array(w222, w221, w220, w219, w218) -> (→"(d) Phase after LabVIEW's unwrapping":dbl[][])
            n177 = Reciprocal(x="Average Size") -> (1/x=w239:dbl)
            n178 = Reciprocal(x="Average Size") -> (1/x=w310:dbl)
            n179 = Reciprocal(x="Average Size") -> (1/x=w243:dbl)
            n180 = Reciprocal(x="Average Size") -> (1/x=w235:dbl)
            n181 = Reciprocal(x="Average Size") -> (1/x=w231:dbl)
            n182 = Reciprocal(x="Average Size") -> (1/x=w192:dbl)
            n183 = Reciprocal(x="Average Size") -> (1/x=w190:dbl)
            n184 = Reciprocal(x="Average Size") -> (1/x=w188:dbl)
            n185 = Reciprocal(x="Average Size") -> (1/x=w186:dbl)
            n186 = Reciprocal(x="Average Size") -> (1/x=w184:dbl)
            n187 = Initialize Array(w239, "Average Size") -> (w238:dbl[])
            n188 = Initialize Array(w310, "Average Size") -> (w309:dbl[])
            n189 = Initialize Array(w243, "Average Size") -> (w242:dbl[])
            n190 = Initialize Array(w235, "Average Size") -> (w234:dbl[])
            n191 = Initialize Array(w231, "Average Size") -> (w230:dbl[])
            n192 = Initialize Array(w192, "Average Size") -> (w191:dbl[])
            n193 = Initialize Array(w190, "Average Size") -> (w189:dbl[])
            n194 = Initialize Array(w188, "Average Size") -> (w187:dbl[])
            n195 = Initialize Array(w186, "Average Size") -> (w185:dbl[])
            n196 = Initialize Array(w184, "Average Size") -> (w183:dbl[])
            n197 = Build Array(w254, w253, w252, w251, w250) -> (→"(e) Phase after LabVIEW's unwrapping + median":dbl[][])
            n198 = call-poly <vilib>:"FIR Filter.vi"("FIR Coefficients"=w238, "X"=w236) -> ("Filtered X"=w225:dbl[])  [unwired: 2 in, 1 out]
            n199 = call-poly <vilib>:"FIR Filter.vi"("FIR Coefficients"=w309, "X"=w307) -> ("Filtered X"=w227:dbl[])  [unwired: 2 in, 1 out]
            n200 = call-poly <vilib>:"FIR Filter.vi"("FIR Coefficients"=w242, "X"=w240) -> ("Filtered X"=w226:dbl[])  [unwired: 2 in, 1 out]
            n201 = call-poly <vilib>:"FIR Filter.vi"("FIR Coefficients"=w234, "X"=w232) -> ("Filtered X"=w224:dbl[])  [unwired: 2 in, 1 out]
            n202 = call-poly <vilib>:"FIR Filter.vi"("FIR Coefficients"=w230, "X"=w228) -> ("Filtered X"=w223:dbl[])  [unwired: 2 in, 1 out]
            n203 = call-poly <vilib>:"FIR Filter.vi"("FIR Coefficients"=w191, "X"=w181) -> ("Filtered X"=w176:dbl[])  [unwired: 2 in, 1 out]
            n204 = call-poly <vilib>:"FIR Filter.vi"("FIR Coefficients"=w189, "X"=w180) -> ("Filtered X"=w175:dbl[])  [unwired: 2 in, 1 out]
            n205 = call-poly <vilib>:"FIR Filter.vi"("FIR Coefficients"=w187, "X"=w179) -> ("Filtered X"=w174:dbl[])  [unwired: 2 in, 1 out]
            n206 = call-poly <vilib>:"FIR Filter.vi"("FIR Coefficients"=w185, "X"=w178) -> ("Filtered X"=w173:dbl[])  [unwired: 2 in, 1 out]
            n207 = call-poly <vilib>:"FIR Filter.vi"("FIR Coefficients"=w183, "X"=w177) -> ("Filtered X"=w172:dbl[])  [unwired: 2 in, 1 out]
            n208 = Build Array(w215, w214, w213, w212, w211) -> (→"(g) Phase after Denpose's unwrapping":dbl[][])
            n209 = Build Array(w203, w202, w201, w200, w199) -> (→"(h) Phase after Denpose unwrapping + median":dbl[][])
            n210 = Build Array(w227, w226, w225, w224, w223) -> (→"(f) Phase after LabVIEW's unwrapping + filters":dbl[][])
            n211 = Build Array(w176, w175, w174, w173, w172) -> (→"(i) Phase of Denpose's processing":dbl[][])
          }
        }
        n212 = local read "OFF"() -> (w122:bool)
        n213 = Compound Arithmetic op=OR(w127, w122, w123) -> (w126:bool)
      }
      n214 = call <instrlib>:"niUSRP Abort.vi"("session handle"=w90, "error in (no error)"=w91) -> ("session handle out"=w89:refnum<k15>, "error out"=w88:errorcluster)  [unwired: 12 in]
      n215 = call <instrlib>:"niUSRP Close Session.vi"("session handle"=w89, "error in (no error)"=w88) -> ("error out"=w86:errorcluster)  [unwired: 13 in]
      n216 = Merge Errors(w86) -> (w85:errorcluster)
    }
    frame Error {
      n217 = local write "ERROR"(TRUE) -> ()
    }
  }
  "receiver error" <- w34
